vi "UpdateRunNumber.vi"(11 "RVCLibrary_Bug2 in":refnum<class "RVCLibrary_Bug2.lvclass">) -> (3 "RVCLibrary_Bug2 out":refnum<class "RVCLibrary_Bug2.lvclass">)   [LabVIEW 2013, in "RVCLibrary_Bug2.lvclass"]
uses:
  RVCLibrary_Bug2.lvclass
  RVCLibrary_Bug2.lvclass/RVCLibrary_Bug2.ctl
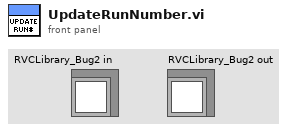
[diagram p1: front panel]
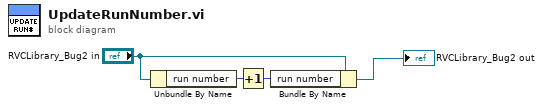
[diagram p0: block diagram]
diagram:
  n1 = Unbundle By Name("RVCLibrary_Bug2 in") -> ("run number"=w3:i32)
  n2 = Increment(x=w3) -> (x+1=w4:i32)
  n3 = Bundle By Name(cluster="RVCLibrary_Bug2 in", "run number"=w4) -> (→"RVCLibrary_Bug2 out":refnum<class "RVCLibrary_Bug2.lvclass">)
